vi "Initialize.vi"(6 "Reset (True)":bool=TRUE, 7 "ID Query (True)":bool=TRUE, 8 "error in (no error)":errorcluster, 10 "Serial Configuration":T1={"Baud Rate (115200)"=115200, "Parity (0: None)"=0, "Data Bits (8)"=8, "Stop Bits (2.0)"=10} {"Stop Bits (2.0)" items=["1.0"=10, "2.0"=20]; "Data Bits (8)" items=["7"=7, "8"=8]; "Parity (0: None)" items=["None", "Odd", "Even"]; "Baud Rate (115200)" items=["4800"=4800, "9600"=9600, "19200"=19200, "57600"=57600, "115200"=115200]}, 11 "VISA resource name":refnum<visa-resource-name>) -> (0 "error out":errorcluster, 3 "VISA resource name out":refnum<visa-resource-name>)   [LabVIEW 2021, in "HH PLI Series.lvlib"]
doc: "Establishes communication with the instrument and optionally performs an instrument identification query and/or an instrument reset. It also places the instrument in a default state needed for other instrument driver operations. Therefore, call this VI before calling other instrument driver VIs for this instrument. Generally, you need to call the Initialize VI only once at the beginning of an application.\n\n<b>VISA resource name examples:</b>\n<b>GPIB:</b> GPIB::7::INSTR\n<b>Serial:</b> COM1\n<b>TCPIP (Socket):</b> TCPIP::192.168.111.100::1001::SOCKET"
uses:
  HH PLI Series.lvlib
panel:
  # "(c) 2013-2015 Hoecherl&Hackl GmbH.  ALL RIGHTS RESERVED."
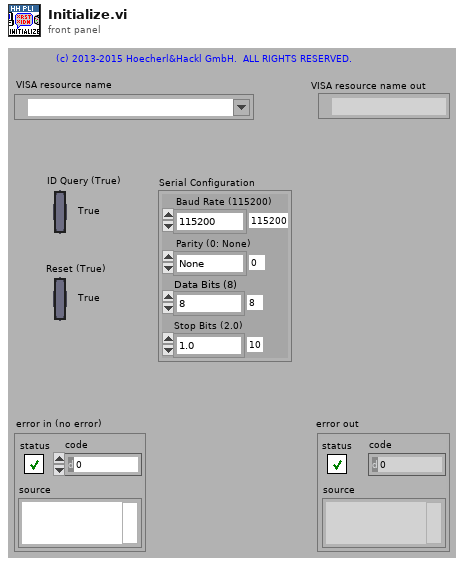
[diagram p1: front panel]
types:
  T1 = cluster{"Baud Rate (115200)":u32, "Parity (0: None)":u16, "Data Bits (8)":u16, "Stop Bits (2.0)":u16}
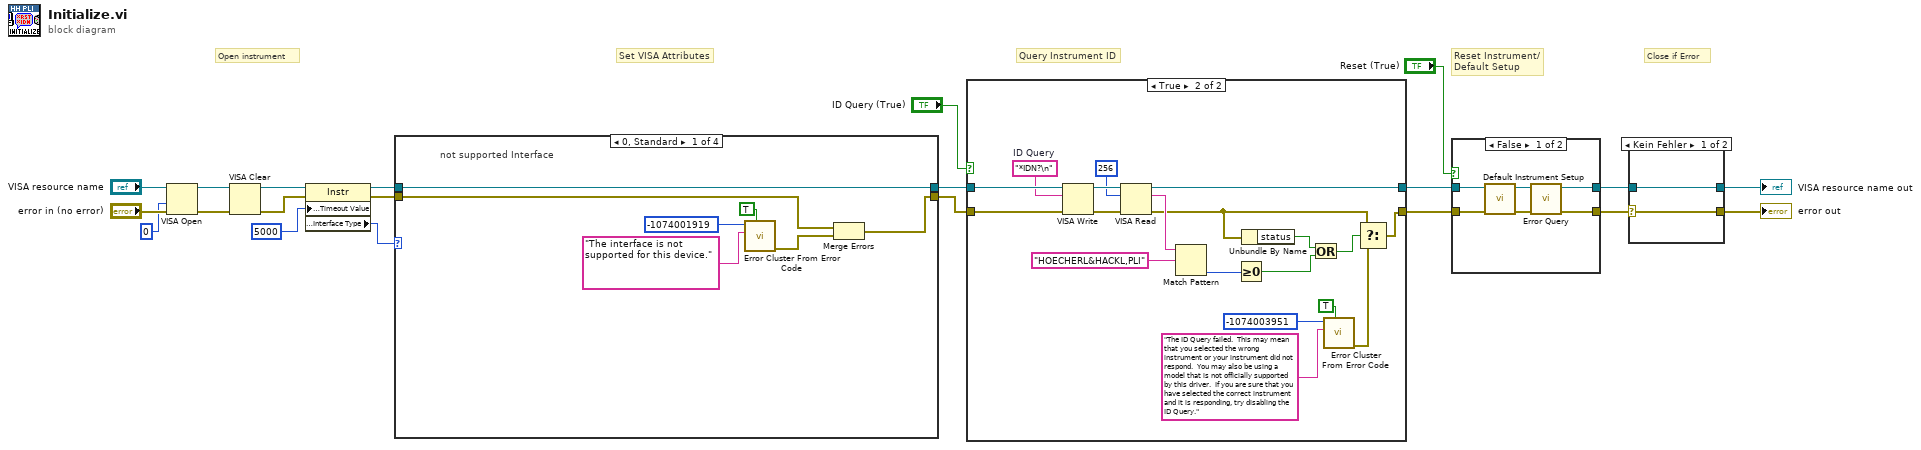
[diagram p0: block diagram]
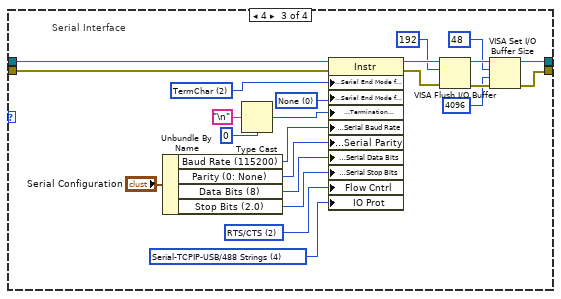
[diagram p3: hidden frame]
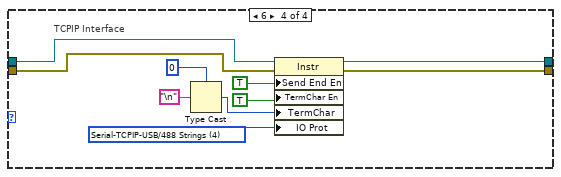
[diagram p4: hidden frame]
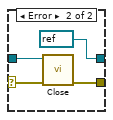
[diagram p5: hidden frame]
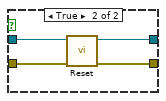
[diagram p6: hidden frame]
diagram:
  # "Set VISA Attributes"
  # "Close if Error"
  # "Query Instrument ID"
  # "Reset Instrument/\nDefault Setup"
  # "Open instrument"
  n1 = VISA Open(access mode=u32 0, error in (no error)="error in (no error)", VISA resource name="VISA resource name") -> (VISA resource name=w9:refnum<visa-resource-name>, error out=w8:errorcluster)  [unwired: 2 in]
  n2 = VISA Clear(VISA resource name=w9, error in (no error)=w8) -> (VISA resource name out=w7:refnum<visa-resource-name>, error out=w6:errorcluster)
  n3 = property class="Instr"(reference=w7, error in=w6, "General Settings:Timeout Value"=u32 5000) -> (reference out=w12:refnum<visa-resource-name>, error out=w11:errorcluster, "Interface Information:Interface Type"=w1:u16)
  n4 = case shown="0, Standard" w1 {
    tunnel: [w28 w30 w50 w61] -> w14
    tunnel: [w24 w29 w47 w60] -> w13
    tunnel: w12 -> [w28 w30 w52 w63]
    tunnel: w11 -> [w23 w29 w53 w62]
    frame 0, Default {
      # "not supported Interface"
      n5 = call <vilib>:"Error Cluster From Error Code.vi"("show call chain? (False)"=TRUE, "error message (\"\")"="The interface is not supported for this device." ("Source (VI Name)"), "error code (0)"=-1074001919 ("Code")) -> ("error out"=w22:errorcluster)  [unwired: 6 in]
      n6 = Merge Errors(w23, w22) -> (w24:errorcluster)
    }
    frame 1 {
      # "GPIB Interface"
    }
    frame 4 {
      w31 = u16 4 items=["Normal"=1, "VXI/FDC"=2, "GPIB/HS488"=3, "Serial-TCPIP-USB/488 Strings"=4, "USBTMC/Vendor-Specific"=5] ("Message Based Settings:IO Protocol")
      w32 = u16 0 items=["None", "Last Bit", "TermChar", "Break"] ("Serial Settings:End Mode for Writes")
      w33 = u16 2 items=["None", "XON/XOFF", "RTS/CTS", "XON/XOFF & RTS/CTS", "DTR/DSR", "XON/XOFF & DTR/DSR"] ("Serial Settings:Flow Control")
      w40 = u16 2 items=["None", "LastBit", "TermChar"] ("Serial Settings:Serial End Mode for Reads")
      # "Serial Interface"
      n7 = Unbundle By Name("Serial Configuration") -> ("Baud Rate (115200)"=w38:u32, "Parity (0: None)"=w36:u16, "Data Bits (8)"=w37:u16, "Stop Bits (2.0)"=w34:u16)
      n8 = Type Cast(type=u8 0, x="\n" ("Line Feed Constant")) -> (*(type *) &x=w39:u8)
      n9 = property class="Instr"(reference=w52, error in=w53, "Serial Settings:Serial End Mode for Reads"=w40, "Serial Settings:Serial End Mode for Writes"=w32, "Message Based Settings:Termination Character"=w39, "Serial Settings:Serial Baud Rate"=w38, "Serial Settings:Serial Parity"=w36, "Serial Settings:Serial Data Bits"=w37, "Serial Settings:Serial Stop Bits"=w34, "Flow Cntrl"=w33, "IO Prot"=w31) -> (reference out=w46:refnum<visa-resource-name>, error out=w49:errorcluster)
      n10 = VISA Flush I/O Buffer(VISA resource name=w46, mask (16)=u16 192, error in (no error)=w49) -> (VISA resource name out=w51:refnum<visa-resource-name>, error out=w48:errorcluster)
      n11 = VISA Set I/O Buffer Size(VISA resource name=w51, mask (16)=u16 48, size (4096)=u32 4096 ("size (0)"), error in (no error)=w48) -> (VISA resource name out=w50:refnum<visa-resource-name>, error out=w47:errorcluster)
    }
    frame 6 {
      w56 = u16 4 items=["Normal"=1, "VXI/FDC"=2, "GPIB/HS488"=3, "Serial-TCPIP-USB/488 Strings"=4, "USBTMC/Vendor-Specific"=5] ("Message Based Settings:IO Protocol")
      # "TCPIP Interface"
      n12 = Type Cast(type=u8 0, x="\n" ("Line Feed Constant")) -> (*(type *) &x=w57:u8)
      n13 = property class="Instr"(reference=w63, error in=w62, "Send End En"=TRUE ("Message Based Settings:Send End Enable"), "TermChar En"=TRUE ("Message Based Settings:Termination Character Enable"), "TermChar"=w57, "IO Prot"=w56) -> (reference out=w61:refnum<visa-resource-name>, error out=w60:errorcluster)
    }
  }
  n14 = case shown="True" "ID Query (True)" {
    tunnel: [w64 w84] -> w20
    tunnel: [w65 w81] -> w21
    tunnel: w14 -> [w65 w82]
    tunnel: w13 -> [w64 w83]
    frame False {
    }
    frame True {
      w75 = "*IDN?\n"  # ID Query
      n15 = VISA Write(VISA resource name=w82, write buffer=w75, error in (no error)=w83) -> (VISA resource name out=w79:refnum<visa-resource-name>, error out=w78:errorcluster)  [unwired: 1 out]
      n16 = VISA Read(VISA resource name=w79, byte count=u32 256, error in (no error)=w78) -> (VISA resource name out=w81:refnum<visa-resource-name>, read buffer=w80:string, error out=w69:errorcluster)  [unwired: 1 out]
      n17 = Match Pattern(string=w80, regular expression="HOECHERL&HACKL,PLI") -> (offset past match=w70:i32)  [unwired: 1 in, 3 out]
      n18 = Greater Or Equal To 0?(x=w70) -> (x >= 0?=w67:bool)
      n19 = Unbundle By Name(w69) -> ("status"=w68:bool)
      n20 = Or(x=w68, y=w67) -> (x .or. y?=w66:bool)
      n21 = call <vilib>:"Error Cluster From Error Code.vi"("show call chain? (False)"=TRUE, "error message (\"\")"="The ID Query failed.  This may mean that you selected the wrong instrument or your instrument did not respond.  You may also be using a model that is not officially supported by this driver.  If you are sure that you have selected the correct instrument and it is responding, try disabling the ID Query." ("Source (VI Name)"), "error code (0)"=-1074003951 ("Code")) -> ("error out"=w74:errorcluster)  [unwired: 6 in]
      n22 = Select(t=w69, s=w66, f=w74) -> (s? t:f=w84:errorcluster)
    }
  }
  n23 = case shown="False" "Reset (True)" {
    tunnel: w20 -> [w89 w91]
    tunnel: [w86 w94] -> w2
    tunnel: w21 -> [w90 w92]
    tunnel: [w87 w93] -> w3
    frame False {
      n24 = call "Default Instrument Setup.vi"("error in (no error)"=w89, "VISA resource name"=w90) -> ("error out"=w85:errorcluster, "VISA resource name out"=w88:refnum<visa-resource-name>)  [unwired: 8 in]
      n25 = call "Error Query.vi"("error in (no error)"=w85, "VISA resource name"=w88) -> ("error out"=w86:errorcluster, "VISA resource name out"=w87:refnum<visa-resource-name>)  [unwired: 6 in, 2 out]
    }
    frame True {
      n26 = call "Reset.vi"("error in (no error)"=w91, "VISA resource name"=w92) -> ("error out"=w94:errorcluster, "VISA resource name out"=w93:refnum<visa-resource-name>)  [unwired: 8 in]
    }
  }
  n27 = case shown="Kein Fehler" w2 {
    selector: w2 -> [w95 w98]
    tunnel: w3 -> [w96 w99]
    tunnel: [w96 refnum<visa-resource-name> refnum ("VISA resource name out")] -> w5
    tunnel: [w95 w100] -> w4
    frame No Error {
    }
    frame Error {
      n28 = call "Close.vi"("error in (no error)"=w98, "VISA resource name"=w99) -> ("error out"=w100:errorcluster)  [unwired: 9 in]
    }
  }
  "VISA resource name out" <- w5
  "error out" <- w4
